vi "DC Motor Speed wo Controller.vi"() -> ()   [LabVIEW 2016]
panel:
  in  "Stop Button":bool
  out "Transient Response with Unit Step Signal as Input":dbl(graph)
  in  "Motor constant":dbl
  in  "moment of inertia of the rotor (kgm^2)":dbl
  in  "Motor viscous friction constant (Nms)":dbl
  in  "Inductance (henry)":dbl
  in  "Resistance (ohm)":dbl
  # "Transient Response of DC Motor Speed (without PID Controller)"
  # "Sourse : http://ctms.engin.umich.edu/CTMS/index.php?example=MotorSpeed&section=SystemAnalysis"
  # "DC Motor Circuit :"
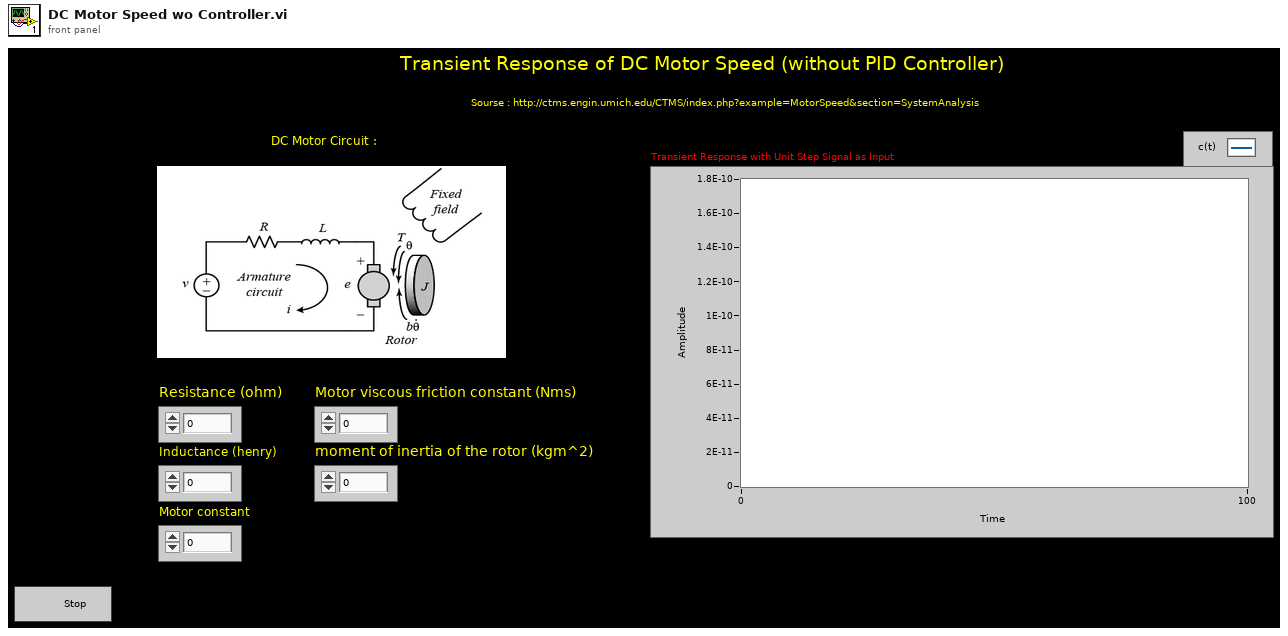
[diagram p1: front panel]
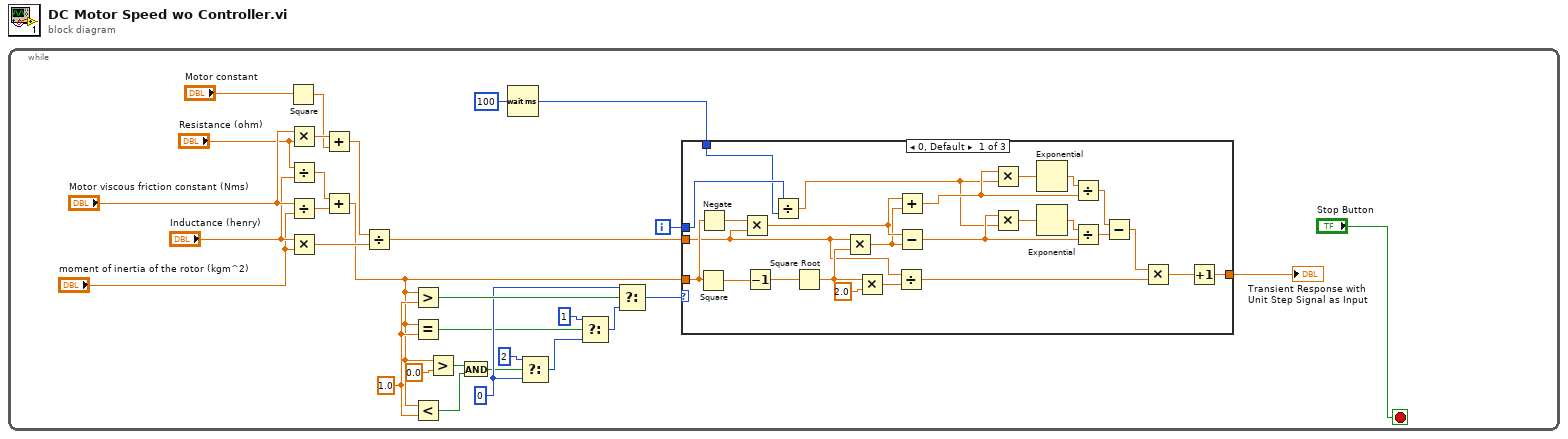
[diagram p0: block diagram]
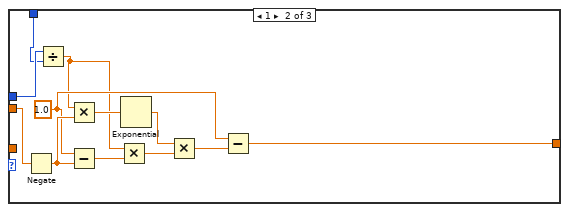
[diagram p2: hidden frame]
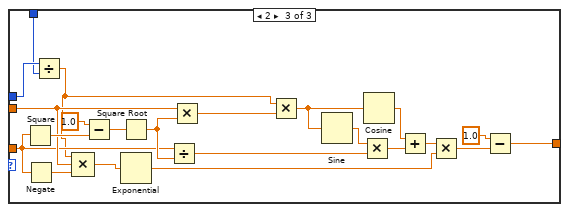
[diagram p3: hidden frame]
diagram:
  n1 = while {
    i -> [w2]
    stop <- "Stop Button" stop-if-true
    w21 = 1.0 ("y")
    w23 = 0
    n2 = Square(x="Motor constant") -> (x^2=w13:dbl)
    n3 = Multiply(x="Motor viscous friction constant (Nms)", y="Resistance (ohm)") -> (x*y=w14:dbl)
    n4 = Divide(x="Resistance (ohm)", y="Inductance (henry)") -> (x/y=w31:dbl)
    n5 = Divide(x="Motor viscous friction constant (Nms)", y="moment of inertia of the rotor (kgm^2)") -> (x/y=w30:dbl)
    n6 = Multiply(x="Inductance (henry)", y="moment of inertia of the rotor (kgm^2)") -> (x*y=w8:dbl)
    n7 = Add(x=w14, y=w13) -> (x+y=w10:dbl)
    n8 = Add(x=w31, y=w30) -> (x+y=w7:dbl)
    n9 = Divide(x=w10, y=w8) -> (x/y=w6:dbl)
    n10 = Greater?(x=w7, y=w21) -> (0:w26:bool)
    n11 = Equal?(x=w7, y=w21) -> (x = y?=w22:bool)
    n12 = Less?(x=w7, y=w21) -> (x < y?=w18:bool)
    n13 = Greater?(x=w7, y=0.0) -> (0:w19:bool)
    n14 = And(x=w19, y=w18) -> (x .and. y?=w17:bool)
    n15 = Wait (ms)(milliseconds to wait=u32 100) -> (millisecond timer value=w1:u32)
    n16 = Select(t=2, s=w17, f=w23) -> (s? t:f=w25:i32)
    n17 = Select(t=1, s=w22, f=w25) -> (s? t:f=w28:i32)
    n18 = Select(t=w23, s=w26, f=w28) -> (s? t:f=w29:i32)
    n19 = case shown="0, Default" w29 {
      tunnel: w7 -> [w55 _ w78]
      tunnel: w6 -> [w39 w68 w80]
      tunnel: [w35 w60 w72] -> w5
      tunnel: w2 -> [w34 w59 w71]
      tunnel: w1 -> [w32 w58 w70]
      frame 0, Default {
        n20 = Square(x=w55) -> (x^2=w54:dbl)
        n21 = Negate(x=w55) -> (-x=w56:dbl)
        n22 = Multiply(x=w56, y=w39) -> (x*y=w52:dbl)
        n23 = Decrement(x=w54) -> (x-1=w53:dbl)
        n24 = Divide(x=w34, y=w32) -> (x/y=w33:dbl)
        n25 = Square Root(x=w53) -> (sqrt(x)=w42:dbl)
        n26 = Multiply(x=w39, y=w42) -> (x*y=w51:dbl)
        n27 = Multiply(x=w42, y=2.0) -> (x*y=w40:dbl)
        n28 = Divide(x=w39, y=w40) -> (x/y=w37:dbl)
        n29 = Add(x=w52, y=w51) -> (x+y=w47:dbl)
        n30 = Subtract(x=w52, y=w51) -> (x-y=w45:dbl)
        n31 = Multiply(x=w47, y=w33) -> (x*y=w50:dbl)
        n32 = Multiply(x=w45, y=w33) -> (x*y=w49:dbl)
        n33 = Exponential(1:w50) -> (0:w48:dbl)
        n34 = Exponential(1:w49) -> (0:w46:dbl)
        n35 = Divide(x=w48, y=w47) -> (x/y=w44:dbl)
        n36 = Divide(x=w46, y=w45) -> (x/y=w43:dbl)
        n37 = Subtract(x=w44, y=w43) -> (x-y=w38:dbl)
        n38 = Multiply(x=w38, y=w37) -> (x*y=w36:dbl)
        n39 = Increment(x=w36) -> (x+1=w35:dbl)
      }
      frame 1 {
        w61 = 1.0 ("x")
        n40 = Negate(x=w68) -> (-x=w67:dbl)
        n41 = Divide(x=w59, y=w58) -> (x/y=w57:dbl)
        n42 = Multiply(x=w57, y=w67) -> (x*y=w65:dbl)
        n43 = Subtract(x=w61, y=w67) -> (x-y=w66:dbl)
        n44 = Multiply(x=w57, y=w66) -> (x*y=w63:dbl)
        n45 = Exponential(1:w65) -> (0:w64:dbl)
        n46 = Multiply(x=w64, y=w63) -> (x*y=w62:dbl)
        n47 = Subtract(x=w61, y=w62) -> (x-y=w60:dbl)
      }
      frame 2 {
        n48 = Square(x=w78) -> (x^2=w90:dbl)
        n49 = Negate(x=w78) -> (-x=w79:dbl)
        n50 = Divide(x=w71, y=w70) -> (x/y=w69:dbl)
        n51 = Compound Arithmetic op=MULTIPLY(w69, w80, w79) -> (w77:dbl)
        n52 = Subtract(x=1.0, y=w90) -> (x-y=w88:dbl)
        n53 = Square Root(x=w88) -> (sqrt(x)=w86:dbl)
        n54 = Exponential(1:w77) -> (0:w75:dbl)
        n55 = Divide(x=w78, y=w86) -> (x/y=w83:dbl)
        n56 = Multiply(x=w80, y=w86) -> (x*y=w87:dbl)
        n57 = Multiply(x=w69, y=w87) -> (x*y=w85:dbl)
        n58 = Sine(x=w85) -> (sin(x)=w84:dbl)
        n59 = Multiply(x=w84, y=w83) -> (x*y=w81:dbl)
        n60 = Cosine(x=w85) -> (cos(x)=w82:dbl)
        n61 = Add(x=w82, y=w81) -> (x+y=w76:dbl)
        n62 = Multiply(x=w76, y=w75) -> (x*y=w74:dbl)
        n63 = Subtract(x=1.0, y=w74) -> (x-y=w72:dbl)
      }
    }
    "Transient Response with Unit Step Signal as Input" <- w5
  }
